vi "View Selected Inverter Parameter Values.vi"(9 "Caller VI Refnum (Callee's Caller)":refnum<vi>, 10 "Inverter v2":T1 {"last updated" format="%<%H:%M\n%d/%m/%Y>T"; "set flag" items=["False", "True"]}) -> ()   [LabVIEW 2019, in "Main.lvclass"]
uses:
  Main.lvclass
  Common/DataTypes/inverter gain range--cluster.ctl
  Common/DataTypes/inverter offset range--cluster.ctl
  Common/DataTypes/inverter info v2--cluster.ctl
  Common/DataTypes/Inverter database record v2--cluster.ctl
panel:
  in  "Close":bool
  out "Selected Inverter":string[][](table)=[["name"], ["last updated"], ["type"], ["inverter Info.manufacturer"], ["inverter Info.model"], ["inverter Info.product"], ["inverter Info.serial"], ["inverter Info.power class"], ["inverter Info.year manf"], ["gain range.max"], ["gain range.min"], ["gain range.increment"], ["offset range.max"], ["offset range.min"], ["offset range.increment"], ["gain actual"], ["offset actual"], ["power level"], ["minimum current"], ["resistance single phase"], ["resistance 3 phase"], ["set flag"]]
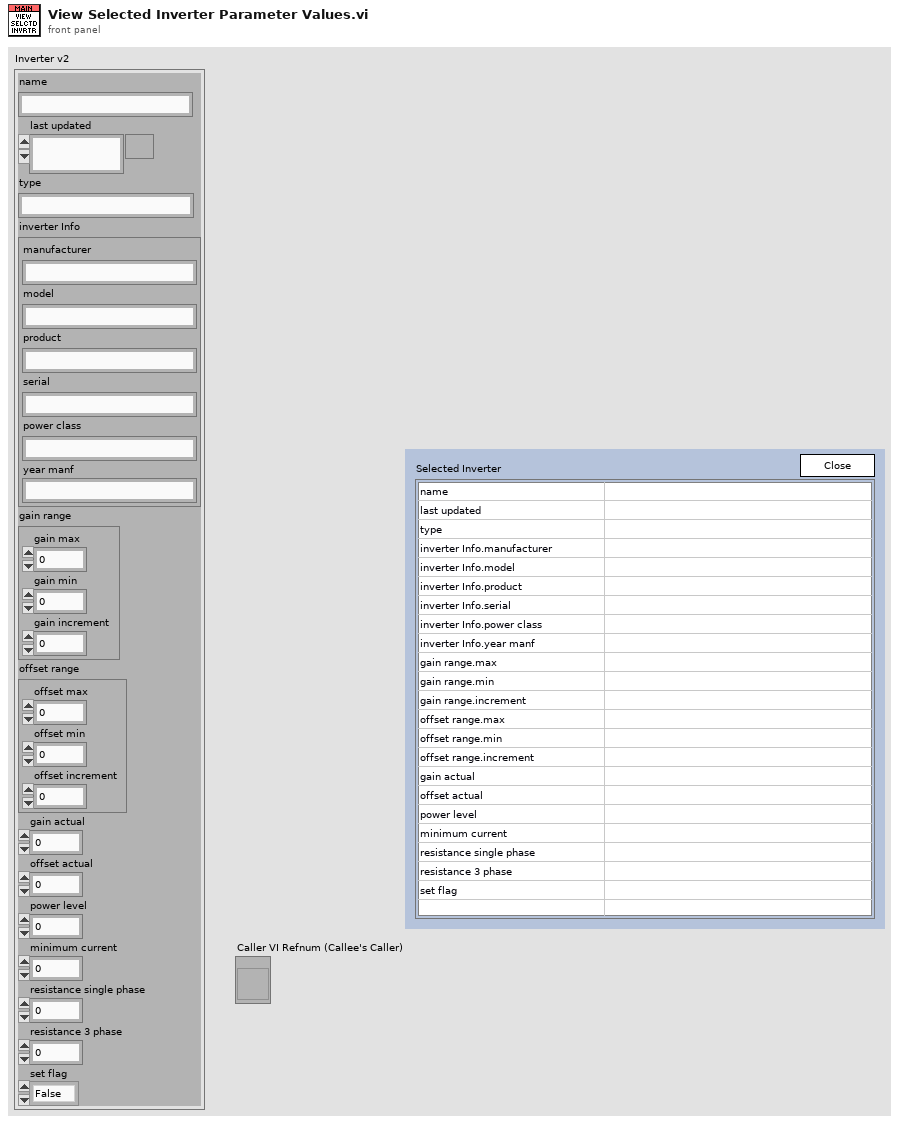
[diagram p1: front panel]
types:
  T1 = typedef "Inverter database record v2--cluster.ctl" = cluster{"name":string, "last updated":timestamp, "type":string, "inverter Info":T2, "gain range":T3, "offset range":T4, "gain actual":dbl, "offset actual":dbl, "power level":dbl, "minimum current":dbl, "resistance single phase":dbl, "resistance 3 phase":dbl, "set flag":u16}
  T2 = typedef "inverter info v2--cluster.ctl" = cluster{"manufacturer":string, "model":string, "product":string, "serial":string, "power class":string, "year manf":string}
  T3 = typedef "inverter gain range--cluster.ctl" = cluster{"gain max":dbl, "gain min":dbl, "gain increment":dbl}
  T4 = typedef "inverter offset range--cluster.ctl" = cluster{"offset max":dbl, "offset min":dbl, "offset increment":dbl}
  T5 = enum32{"Invalid", "Default", "Floating", "Floating/Auto-Hide", "Modal"}
  T6 = enum32{"Invalid", "Standard", "Closed", "Hidden", "Minimized", "Maximized"}
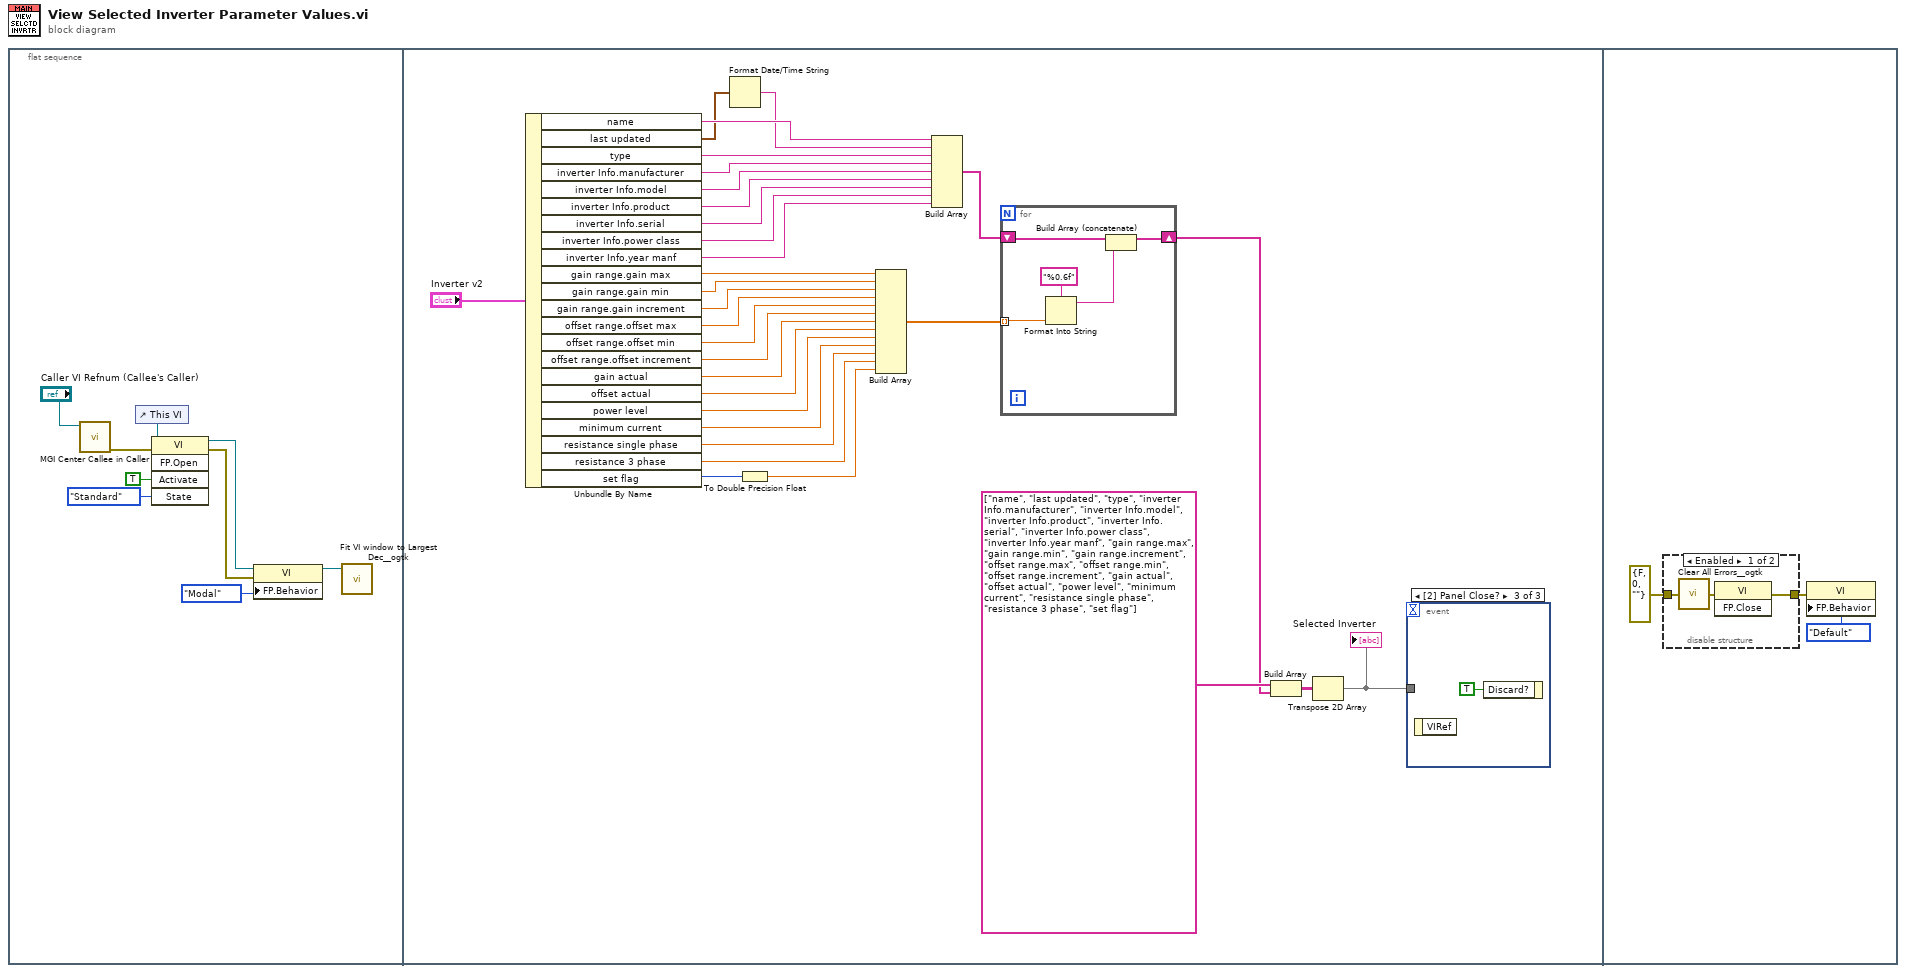
[diagram p0: block diagram]
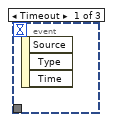
[diagram p2: hidden frame]
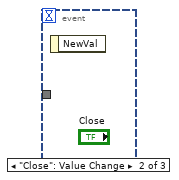
[diagram p3: hidden frame]
diagram:
  n1 = flat-sequence {
    frame #0 {
      n2 = call <userlib>:"MGI Center Callee in Caller.vi"("Caller VI Refnum (Callee's Caller)"="Caller VI Refnum (Callee's Caller)") -> ("Error Out"=w3:errorcluster)  [unwired: 10 in]
      n3 = control-ref of="This VI"() -> (w1:refnum<vi>)
      n4 = invoke class="VI" method="FP.Open"(reference=w1, error in=w3, "Activate"=TRUE ("Activate?"), "State"=T6."Standard") -> (reference out=w8:refnum<vi>, error out=w7:errorcluster)  [unwired: 1 in, 3 out]
      n5 = property class="VI"(reference=w8, error in=w7, "FP.Behavior"=T5."Modal" ("Front Panel Window:Behavior")) -> (reference out=w9:refnum<vi>)  [unwired: 1 out]
      n6 = call <userlib>:"Fit VI window to Largest Dec__ogtk.vi"("VI Ref (calling VI)"=w9) -> ()  [unwired: 5 in, 2 out]
    }
    frame #1 {
      n7 = Unbundle By Name("Inverter v2") -> ("name"=w38:string, "last updated"=w11:timestamp, "type"=w37:string, "inverter Info.manufacturer"=w36:string, "inverter Info.model"=w35:string, "inverter Info.product"=w34:string, "inverter Info.serial"=w33:string, "inverter Info.power class"=w32:string, "inverter Info.year manf"=w12:string, "gain range.gain max"=w31:dbl, "gain range.gain min"=w30:dbl, "gain range.gain increment"=w29:dbl, "offset range.offset max"=w28:dbl, "offset range.offset min"=w27:dbl, "offset range.offset increment"=w26:dbl, "gain actual"=w25:dbl, "offset actual"=w24:dbl, "power level"=w23:dbl, "minimum current"=w22:dbl, "resistance single phase"=w21:dbl, "resistance 3 phase"=w20:dbl, "set flag"=w19:u16)
      n8 = Format Date/Time String(seconds (now)=w11) -> (date/time string=w10:string)  [unwired: 2 in]
      n9 = To Double Precision Float(number=w19) -> (double precision float=w16:dbl)
      n10 = Build Array(w31, w30, w29, w28, w27, w26, w25, w24, w23, w22, w21, w20, w16) -> (w17:dbl[])
      n11 = Build Array(w38, w10, w37, w36, w35, w34, w33, w32, w12) -> (w18:string[])
      n12 = for {
        shift-right: [w41] -> w15
        shift-left: w18 -> [w45]
        tunnel: w17 -> [w44] mode=indexing
        n13 = Format Into String(format string="%0.6f", w44) -> (resulting string=w42:string)  [unwired: 2 in, 1 out]
        n14 = Build Array (concatenate)(w45, w42) -> (w41:string[])
      }
      n15 = Build Array(string[] ["name", "last updated", "type", "inverter Info.manufacturer", "inverter Info.model", "inverter Info.product", "inverter Info.serial", "inverter Info.power class", "inverter Info.year manf", "gain range.max", "gain range.min", "gain range.increment", "offset range.max", "offset range.min", "offset range.increment", "gain actual", "offset actual", "power level", "minimum current", "resistance single phase", "resistance 3 phase", "set flag"] ("subarray"), w15) -> (w14:string[][])
      n16 = Transpose 2D Array(2D array=w14) -> (transposed array=w13:string[][])
      "Selected Inverter" <- w13
      n17 = event shown="[2] Panel Close?" {
        selector: _ -> [_ _ _]
        dyn-events: _ -> [_ _ _]
        timeout: _ -> [_ _ _]
        tunnel: w13 -> [_ _ _]
        event Timeout {
          n18 = event-data() -> ()  [unwired: 1 in, 3 out]
        }
        event "Close": Value Change {
          n19 = event-data() -> ()  [unwired: 1 in, 1 out]
        }
        event Panel Close? {
          n20 = event-data() -> ()  [unwired: 1 in, 1 out]
          n21 = event-data("Discard?"=TRUE) -> ()  [unwired: 1 in, 1 out]
        }
      }
    }
    frame #2 {
      n22 = disable-structure shown="Enabled" {
        disable-tunnel: [w52 w53] -> w49
        disable-tunnel: errorcluster {"status"=FALSE, "code"=0, "source"=""} ("Error In") -> [w50 w53]
        frame Enabled {
          n23 = call <userlib>:"Clear All Errors__ogtk.vi"("Error In"=w50) -> ("Error Out"=w51:errorcluster)  [unwired: 3 in]
          n24 = invoke class="VI" method="FP.Close"(error in=w51) -> (error out=w52:errorcluster)  [unwired: 2 in, 2 out]
        }
        frame Disabled {
        }
      }
      n25 = property class="VI"(error in=w49, "FP.Behavior"=T5."Default" ("Front Panel Window:Behavior")) -> ()  [unwired: 1 in, 2 out]
    }
  }
